vi "toMsgUE.vi"(8 "error in":errorcluster, 11 "ITaskChannel":refnum<class "ITaskChannel.lvclass">) -> (0 "error out":errorcluster, 3 "userEventRef":refnum<user-event>)   [LabVIEW 2023, in "TLC_Daemon.lvlib"]
uses:
  TLC_Daemon.lvlib
  MsgUETaskChannel/MsgUETaskChannel.lvclass
  ITaskChannel/ITaskChannel.lvclass
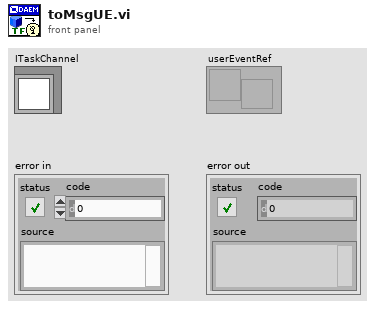
[diagram p1: front panel]
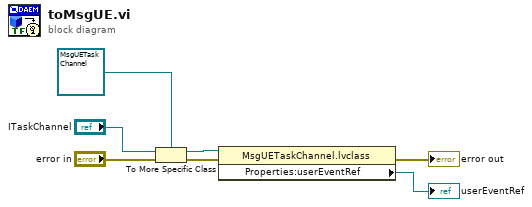
[diagram p0: block diagram]
diagram:
  n1 = To More Specific Class(target class=refnum<class "MsgUETaskChannel.lvclass"> refnum ("TLC_Daemon.lvlib:MsgUETaskChannel.lvclass"), reference="ITaskChannel", error in="error in") -> (specific class reference=w5:refnum<class "MsgUETaskChannel.lvclass">, error out=w6:errorcluster)
  n2 = property class="MsgUETaskChannel.lvclass"(reference=w5, error in=w6) -> (error out=→"error out":errorcluster, "Properties:userEventRef"=→"userEventRef":refnum<user-event>)  [unwired: 1 out]
